vi "getDevice.vi"(8 "error in (no error)":errorcluster, 11 "AdvancedRemote in":refnum<class "AdvancedRemote.lvclass">) -> (0 "error out":errorcluster, 2 "Device.lvclass":refnum<class "Device.lvclass">, 3 "AdvancedRemote out":refnum<class "AdvancedRemote.lvclass">)   [LabVIEW 2017, in "AdvancedRemote.lvclass"]
uses:
  AdvancedRemote.lvclass
  Device Class/Device.lvclass
  AdvancedRemote.lvclass/AdvancedRemote.ctl
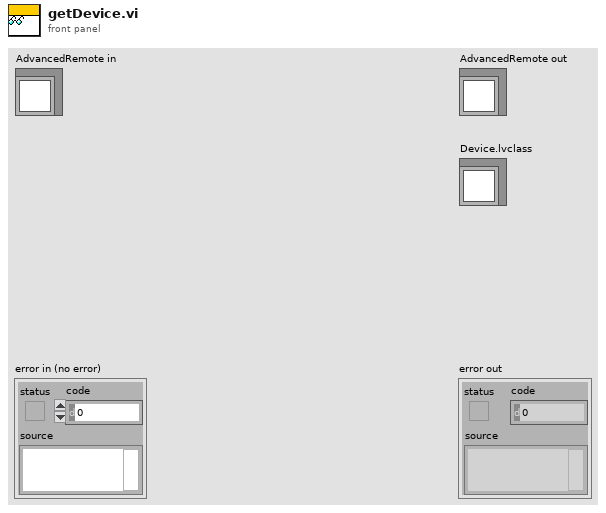
[diagram p1: front panel]
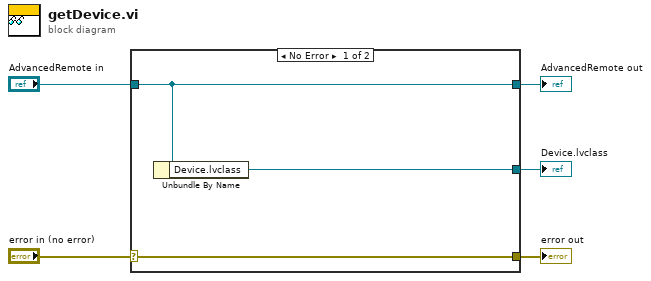
[diagram p0: block diagram]
diagram:
  n1 = case shown="No Error" "error in (no error)" {
    selector: "error in (no error)" -> [w8 w9]
    tunnel: [w8 w9] -> w4
    tunnel: [w7 w10] -> w2
    tunnel: "AdvancedRemote in" -> [w7 w10]
    tunnel: [w6 _] -> w1
    frame No Error {
      n2 = Unbundle By Name(w7) -> ("Device.lvclass"=w6:refnum<class "Device.lvclass">)
    }
    frame Error {
    }
  }
  "error out" <- w4
  "AdvancedRemote out" <- w2
  "Device.lvclass" <- w1
